vi "PSO_CreateNewSwarm.vi"(6 "Parameters":T3={"Swarm size"=100, "Generations no."=500, "Cognitive coeff a1"=6.0, "Social coeff a2"=0.85, "Min inertia weight"=0.0, "Max inertia weight "=0.9, "Fmax"=0} {"Generations no." min=1; "Swarm size" min=1}, 7 "Fitness Function":T2, 8 "Generation":i32, 11 "Population in":T1) -> (3 "Population out":T1)   [LabVIEW 2016, in "Optimal Frequency Bands Search.lvlib" / "ParticleSwarm.lvlib"]
doc: "Рассчитать новые значения координат для частиц роя. Выполнить оценку функции приспособленности для частиц в их новом положении"
uses:
  ParticleSwarm.lvlib
  PSO_tParameters.ctl
  tFitness Function.ctl
  PSO_tPopulation.ctl
panel:
  # "This VI is a part of BCI Design library, http://www.ru-bci.org \nCopyright © 2020, Sotnikov Peter, All rights reserved. License: GNU GPLv3"
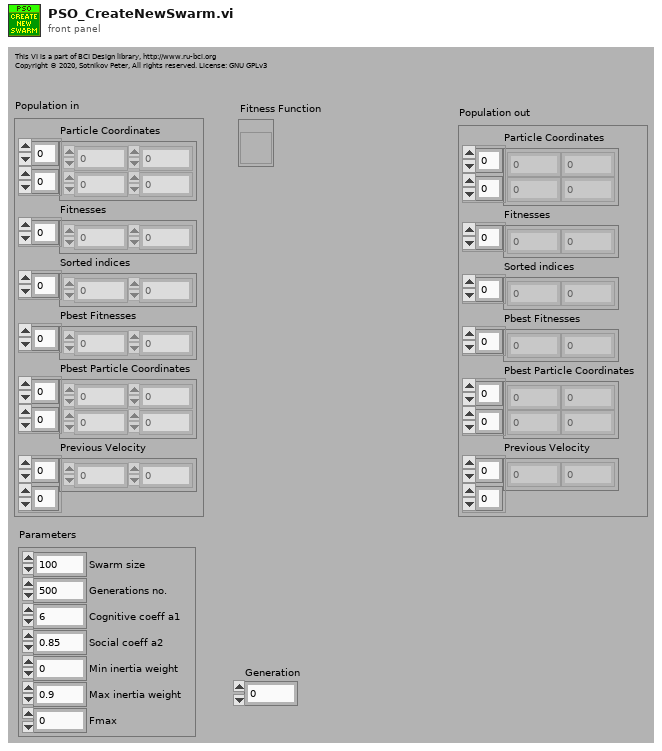
[diagram p1: front panel]
types:
  T1 = typedef "Optimal Frequency Bands Search.lvlib/ParticleSwarm.lvlib/PSO_tPopulation.ctl" = cluster{"Particle Coordinates":i32[][], "Fitnesses":dbl[], "Sorted indices":i32[], "Pbest Fitnesses":dbl[], "Pbest Particle Coordinates":i32[][], "Previous Velocity":dbl[][]}
  T2 = typedef "Optimal Frequency Bands Search.lvlib/ParticleSwarm.lvlib/tFitness Function.ctl" = refnum<vi>
  T3 = typedef "Optimal Frequency Bands Search.lvlib/ParticleSwarm.lvlib/PSO_tParameters.ctl" = cluster{"Swarm size":i32, "Generations no.":i32, "Cognitive coeff a1":dbl, "Social coeff a2":dbl, "Min inertia weight":dbl, "Max inertia weight ":dbl, "Fmax":i32}
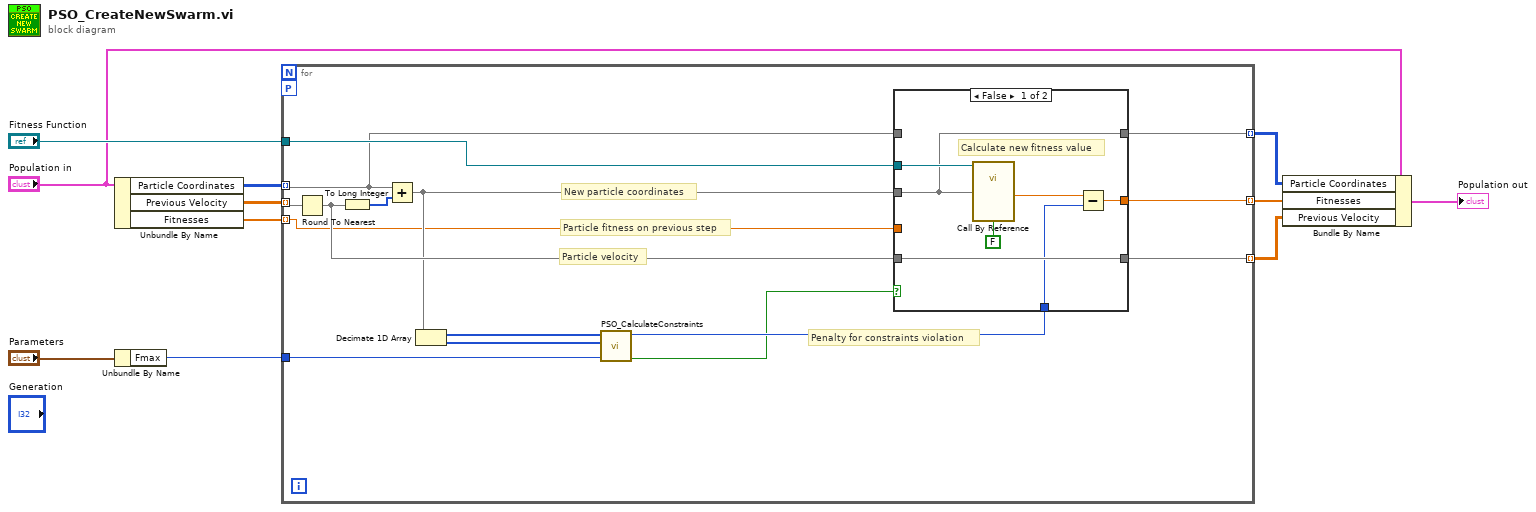
[diagram p0: block diagram]
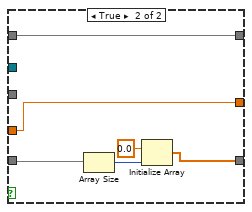
[diagram p2: hidden frame]
diagram:
  n1 = Unbundle By Name("Population in") -> ("Particle Coordinates"=w11:i32[][], "Previous Velocity"=w10:dbl[][], "Fitnesses"=w3:dbl[])
  n2 = Unbundle By Name("Parameters") -> ("Fmax"=w1:i32)
  n3 = for {
    tunnel: w11 -> [w18] mode=indexing
    tunnel: w10 -> [w24] mode=indexing
    tunnel: "Fitness Function" -> [w26]
    tunnel: [w25] -> w4 mode=indexing
    tunnel: [w19] -> w6 mode=indexing
    tunnel: [w22] -> w5 mode=indexing
    tunnel: w3 -> [w17] mode=indexing
    tunnel: w1 -> [w12]
    workers-P: _ -> [_]
    # "Particle fitness on previous step"
    # "New particle coordinates"
    # "Particle velocity"
    # "Penalty for constraints violation"
    n4 = Round To Nearest(number=w24) -> (nearest integer value=w21:dbl[])
    n5 = To Long Integer(number=w21) -> (32bit integer=w23:i32[])
    n6 = Add(x=w18, y=w23) -> (x+y=w20:i32[])
    n7 = Decimate 1D Array(w20) -> (w16:i32[], w15:i32[])
    n8 = call "PSO_CalculateConstraints.vi"("Fmax"=w12, "deltaF vector"=w15, "F0 vector"=w16) -> ("Violation?"=w13:bool, "Penalty"=w14:i32)  [unwired: 7 in]
    n9 = case shown="False" w13 {
      tunnel: w26 -> [w33 _]
      tunnel: [w29 w34] -> w25
      tunnel: [w31 w37] -> w22
      tunnel: w21 -> [w31 w39]
      tunnel: w20 -> [w30 _]
      tunnel: [w30 w35] -> w19
      tunnel: w18 -> [_ w35]
      tunnel: w17 -> [_ w34]
      tunnel: w14 -> [w28 _]
      frame False {
        # "Calculate new fitness value"
        n10 = call-by-ref "Call By Reference"(reference=w33, "Init? (F)"=FALSE, "Phenotype"=w30) -> ("Fitness"=w27:dbl)  [unwired: 2 in, 2 out]
        n11 = Subtract(x=w27, y=w28) -> (x-y=w29:dbl)
      }
      frame True {
        n12 = Array Size(array=w39) -> (size(s)=w38:i32)
        n13 = Initialize Array(0.0 ("Fitness"), w38) -> (w37:dbl[])
      }
    }
  }
  n14 = Bundle By Name(cluster="Population in", "Particle Coordinates"=w6, "Fitnesses"=w4, "Previous Velocity"=w5) -> (→"Population out":T1)
